vi "Get Update Measurement.vi"(8 "Error In":errorcluster, 10 "Waveform Graph In":dynamicdata(graph), 11 "Display Panel V3 In":refnum<class "Display Panel V3.lvclass">) -> (0 "Error Out":errorcluster, 3 "Display Panel V3 Out":refnum<class "Display Panel V3.lvclass">)   [LabVIEW 2014, in "Display Panel.lvlib" / "Display Panel V3.lvclass"]
doc: "This Vi takes the waveform input and convert it to a refnum"
uses:
  Display Panel V3.lvclass
  Display Panel V3.lvclass/Display Panel V3.ctl
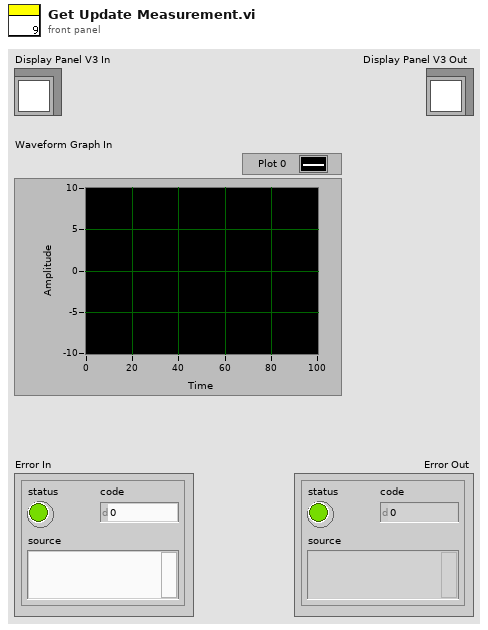
[diagram p1: front panel]
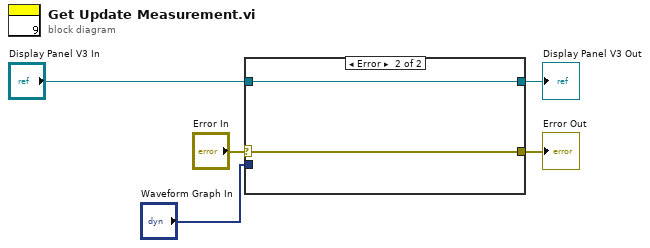
[diagram p0: block diagram]
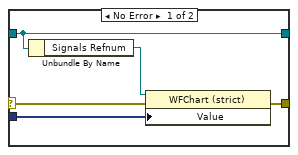
[diagram p2: hidden frame]
diagram:
  n1 = case shown="Error" "Error In" {
    selector: "Error In" -> [w8 w12]
    tunnel: [w7 w12] -> w5
    tunnel: "Display Panel V3 In" -> [w6 w11]
    tunnel: "Waveform Graph In" -> [w9 _]
    tunnel: [w6 w11] -> w2
    frame No Error {
      n2 = Unbundle By Name(w6) -> ("Signals Refnum"=w10:refnum<vi>)
      n3 = property class="WFChart (strict)"(reference=w10, error in=w8, "Value"=w9) -> (error out=w7:errorcluster)  [unwired: 1 out]
    }
    frame Error {
    }
  }
  "Error Out" <- w5
  "Display Panel V3 Out" <- w2
